vi "Add Library and Class Hierarchy Levels.vi"(11 "Hierarchy Array":string[](array[string])) -> (3 "Modified Hierarchy Array":string[](array[string]))   [LabVIEW 2023]
doc: "Modifies <B>Hierarchy Array</B> based on the presence of .lvlib or .lvclass files, and current LabVIEW folder hierarchy standards for those items."
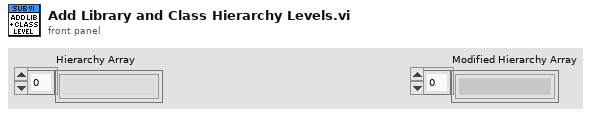
[diagram p1: front panel]
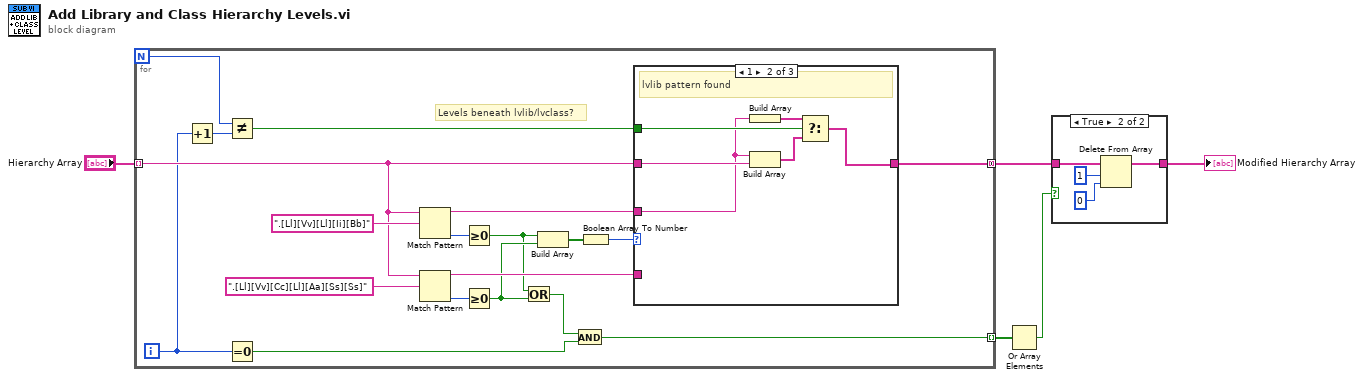
[diagram p0: block diagram]
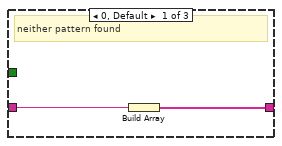
[diagram p3: hidden frame]
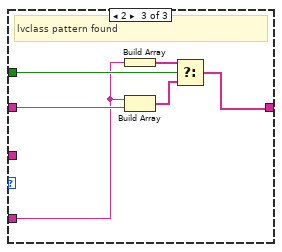
[diagram p4: hidden frame]
diagram:
  n1 = for {
    N -> [w13]
    tunnel: "Hierarchy Array" -> [w18] mode=indexing
    tunnel: [w17] -> w3 mode=concatenating
    tunnel: [w6] -> w4 mode=indexing
    i -> [w11]
    # "Levels beneath lvlib/lvclass?"
    n2 = Increment(x=w11) -> (x+1=w14:i32)
    n3 = Not Equal?(x=w13, y=w14) -> (x != y?=w12:bool)
    n4 = Equal To 0?(x=w11) -> (x = 0?=w10:bool)
    n5 = Match Pattern(string=w18, regular expression=".[Ll][Vv][Ll][Ii][Bb]" ("search string/char (-)")) -> (before substring=w16:string, offset past match=w22:i32)  [unwired: 1 in, 2 out]
    n6 = Match Pattern(string=w18, regular expression=".[Ll][Vv][Cc][Ll][Aa][Ss][Ss]" ("search string/char (-)")) -> (before substring=w15:string, offset past match=w21:i32)  [unwired: 1 in, 2 out]
    n7 = Greater Or Equal To 0?(x=w22) -> (x >= 0?=w8:bool)
    n8 = Greater Or Equal To 0?(x=w21) -> (x >= 0?=w9:bool)
    n9 = Or(x=w8, y=w9) -> (x .or. y?=w7:bool)
    n10 = Build Array(w8, w9) -> (w20:bool[])
    n11 = And(x=w7, y=w10) -> (x .and. y?=w6:bool)
    n12 = Boolean Array To Number(Boolean array=w20) -> (number=w19:u32)
    n13 = case shown="1" w19 {
      tunnel: w18 -> [w26 w32 w38]
      tunnel: [w25 w27 w34] -> w17
      tunnel: w16 -> [_ w29 _]
      tunnel: w15 -> [_ _ w33]
      tunnel: w12 -> [_ w31 w37]
      frame 0, Default {
        # "neither pattern found"
        n14 = Build Array(w26) -> (w25:string[])
      }
      frame 1 {
        # "lvlib pattern found"
        n15 = Build Array(w29) -> (w28:string[])
        n16 = Build Array(w29, w32) -> (w30:string[])
        n17 = Select(t=w28, s=w31, f=w30) -> (s? t:f=w27:string[])
      }
      frame 2 {
        # "lvclass pattern found"
        n18 = Build Array(w33) -> (w35:string[])
        n19 = Build Array(w33, w38) -> (w36:string[])
        n20 = Select(t=w35, s=w37, f=w36) -> (s? t:f=w34:string[])
      }
    }
  }
  n21 = Or Array Elements(Boolean array=w4) -> (logical OR=w2:bool)
  n22 = case shown="True" w2 {
    tunnel: w3 -> [w39 w43]
    tunnel: [w39 w40] -> w1
    frame False {
    }
    frame True {
      n23 = Delete From Array(array=w43, length=1, index=0) -> (array with subset deleted=w40:string[])  [unwired: 1 out]
    }
  }
  "Modified Hierarchy Array" <- w1
